vi "smartHome.vi"(5 "Device in":refnum<k24>) -> (2 "Device out":refnum<k24>)   [LabVIEW 2021]
doc: "André Romero - 2017\nandretec@ifsc.usp.br"
uses:
  C:/user-Lab/AndreTec/GITs/andretec/Thorlabs-Vector-Move/kinesisTec/Kinesis/Thorlabs.MotionControl.TCube.DCServoCLI.dll
  Kinesis/Thorlabs.MotionControl.TCube.DCServoCLI.dll
panel:
  out "array 2":bool[](array[boolean])
  out "array":bool[](array[boolean])
  out "String":string
  out "GetPOS 2":dbl
  out "GetPOS":dbl
  out "new Target":dbl
  out "old Target":dbl
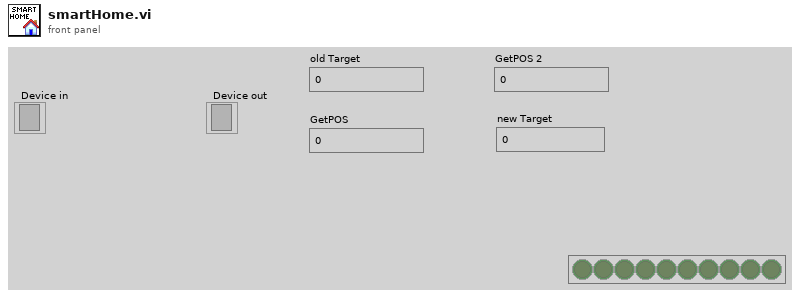
[diagram p1: front panel]
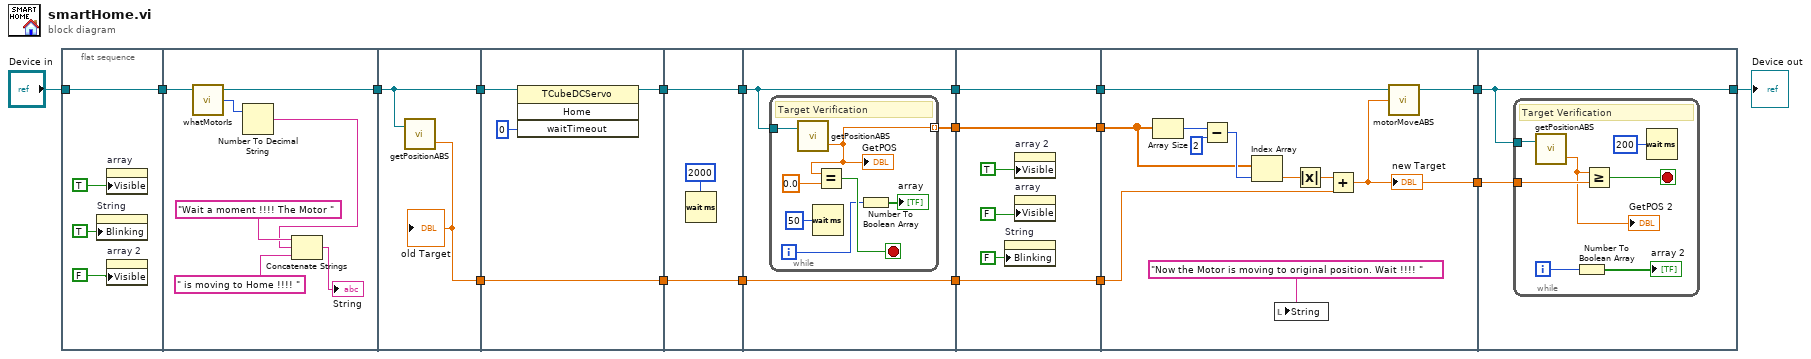
[diagram p0: block diagram]
diagram:
  n1 = flat-sequence {
    tunnel: "Device in" -> [w22]
    tunnel: [w22] -> w1
    tunnel: [w29] -> w8
    tunnel: w1 -> [w28]
    tunnel: [w31] -> w18
    tunnel: [w30] -> w17
    tunnel: w8 -> [w31]
    tunnel: [w34] -> w16
    tunnel: w18 -> [w33]
    tunnel: [w32] -> w15
    tunnel: w17 -> [w32]
    tunnel: [w38] -> w14
    tunnel: w16 -> [w38]
    tunnel: [w36] -> w13
    tunnel: w15 -> [w36]
    tunnel: w14 -> [w40]
    tunnel: [w41] -> w7
    tunnel: [w40] -> w5
    tunnel: w13 -> [w39]
    tunnel: [w39] -> w3
    tunnel: w7 -> [w54]
    tunnel: [w54] -> w6
    tunnel: w5 -> [w53]
    tunnel: [w53] -> w4
    tunnel: w3 -> [w52]
    tunnel: [w52] -> w2
    tunnel: w6 -> [w60]
    tunnel: w4 -> [w58]
    tunnel: w2 -> [w57]
    tunnel: [w59] -> w12
    tunnel: [w56] -> w11
    tunnel: [w67] -> w9
    tunnel: w12 -> [w67]
    tunnel: w11 -> [w66]
    frame #0 {
      n2 = property on="String" class="Str"("Blinking"=TRUE) -> ()  [unwired: 2 in, 2 out]
      n3 = property on="array" class="Arr (strict)"("Visible"=TRUE) -> ()  [unwired: 2 in, 2 out]
      n4 = property on="array 2" class="Arr (strict)"("Visible"=FALSE) -> ()  [unwired: 2 in, 2 out]
    }
    frame #1 {
      n5 = call "whatMotorIs.vi"("Device in"=w28) -> ("SerialNumber"=w27:u32, "Device out"=w29:refnum<k24>)  [unwired: 3 in]
      n6 = Number To Decimal String(number=w27) -> (decimal integer string=w23:string)  [unwired: 1 in]
      n7 = Concatenate Strings("Wait a moment !!!! The Motor ", w23, " is moving to Home !!!! ") -> (→"String":string)
    }
    frame #2 {
      n8 = call "getPositionABS.vi"("Device"=w31) -> ("GetPOS"=w30:dbl)  [unwired: 1 in, 1 out]
      "old Target" <- w30
    }
    frame #3 {
      n9 = invoke class="TCubeDCServo" method="Home"(reference=w33, "waitTimeout"=0) -> (reference out=w34:refnum<k24>)  [unwired: 2 in, 3 out]
    }
    frame #4 {
      n10 = Wait (ms)(milliseconds to wait=u32 2000) -> ()  [unwired: 1 out]
    }
    frame #5 {
      n11 = while {
        tunnel: w40 -> [w48]
        tunnel: [w42] -> w41 mode=indexing
        i -> [w43]
        stop <- w45 stop-if-true
        # "Target Verification"
        n12 = call "getPositionABS.vi"("Device"=w48) -> ("GetPOS"=w42:dbl)  [unwired: 1 in, 1 out]
        "GetPOS" <- w42
        n13 = Wait (ms)(milliseconds to wait=u32 50) -> ()  [unwired: 1 out]
        n14 = Equal?(x=w42, y=0.0) -> (x = y?=w45:bool)
        n15 = Number To Boolean Array(number=w43) -> (Boolean array=→"array":bool[])
      }
    }
    frame #6 {
      n16 = property on="String" class="Str"("Blinking"=FALSE) -> ()  [unwired: 2 in, 2 out]
      n17 = property on="array 2" class="Arr (strict)"("Visible"=TRUE) -> ()  [unwired: 2 in, 2 out]
      n18 = property on="array" class="Arr (strict)"("Visible"=FALSE) -> ()  [unwired: 2 in, 2 out]
    }
    frame #7 {
      n19 = Array Size(array=w60) -> (size(s)=w63:i32)
      n20 = Subtract(x=w63, y=2) -> (x-y=w62:i32)
      n21 = Index Array(array=w60, index=w62) -> (element=w64:dbl)
      n22 = local write "String"("Now the Motor is moving to original position. Wait !!!! ") -> ()
      n23 = Absolute Value(x=w64) -> (abs(x)=w65:dbl)
      n24 = Add(x=w65, y=w57) -> (x+y=w56:dbl)
      "new Target" <- w56
      n25 = call "motorMoveABS.vi"("position"=w56, "Device in"=w58) -> ("Device out"=w59:refnum<k24>)  [unwired: 3 in]
    }
    frame #8 {
      n26 = while {
        tunnel: w67 -> [w73]
        tunnel: w66 -> [w72]
        i -> [w70]
        stop <- w71 stop-if-true
        # "Target Verification"
        n27 = call "getPositionABS.vi"("Device"=w73) -> ("GetPOS"=w68:dbl)  [unwired: 1 in, 1 out]
        "GetPOS 2" <- w68
        n28 = Number To Boolean Array(number=w70) -> (Boolean array=→"array 2":bool[])
        n29 = Greater Or Equal?(x=w68, y=w72) -> (x >= y?=w71:bool)
        n30 = Wait (ms)(milliseconds to wait=u32 200) -> ()  [unwired: 1 out]
      }
    }
  }
  "Device out" <- w9
